vi "TestData_TestAddHash.vi"(8 "error in (no error)":errorcluster caption="错误输入（无错误）", 10 "Record_Text":string, 11 "分隔符(Tab)":string) -> (0 "error out":errorcluster caption="错误输出", 1 "Hash_Code":string, 2 "RecordText Outpout":string, 3 "ok?":bool)   [LabVIEW 2012, in "Lib_UEL.ATE.lvlib" / "Lib_TestData.lvlib"]
uses:
  Lib_TestData.lvlib
  App/Lib_App.lvlib
panel:
  # "功能说明:\n- 添加Hash列\n- 兼容不同的分隔符.\n- 兼容已知的错误格式\n\n\n插入语句标准: 留意转换后最后一列为空.\n- 255列, 以#分隔, \n- 251列, 以#分隔, 缺少: No47记录后,spare1~4列\n- 添加最后一列: hash列"
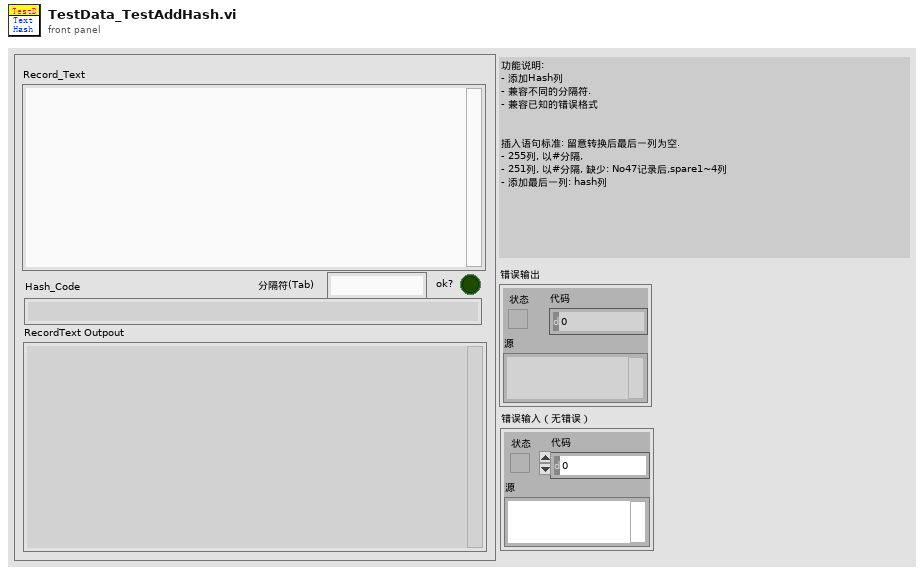
[diagram p1: front panel]
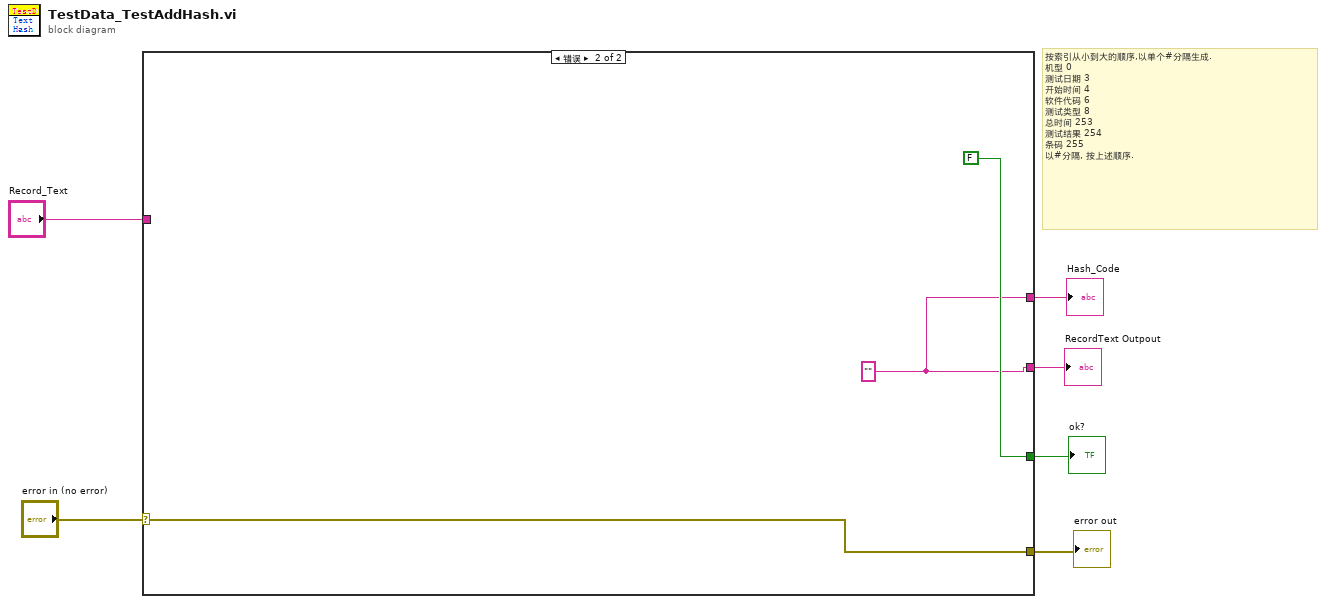
[diagram p0: block diagram]
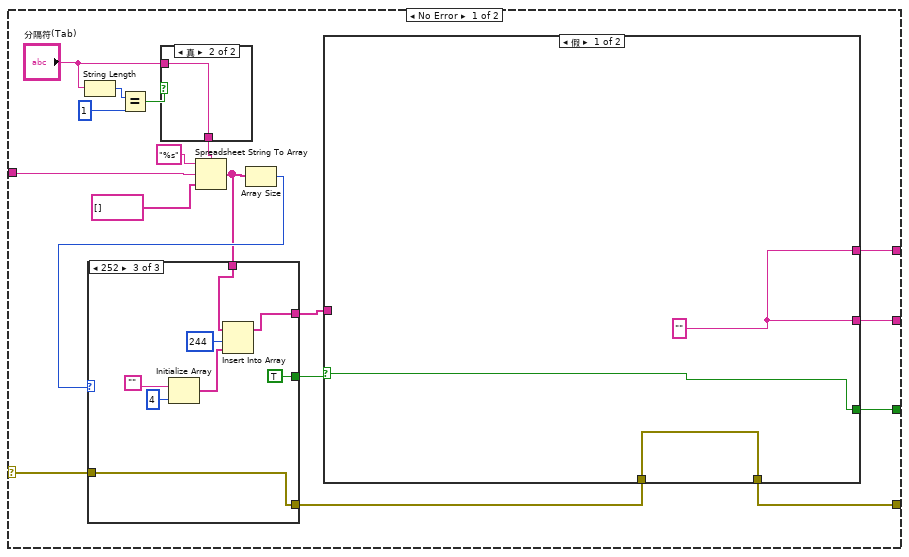
[diagram p2: hidden frame]
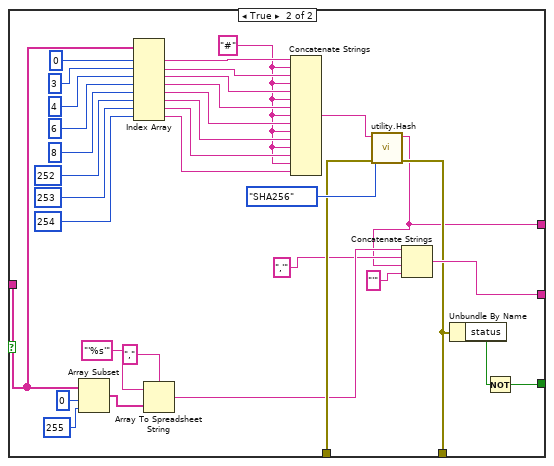
[diagram p3: hidden frame]
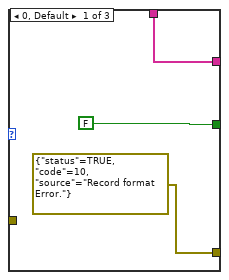
[diagram p4: hidden frame]
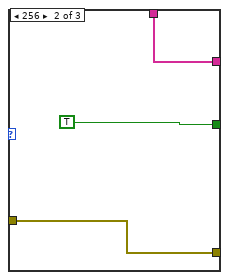
[diagram p5: hidden frame]
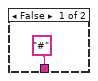
[diagram p6: hidden frame]
diagram:
  # "按索引从小到大的顺序,以单个#分隔生成.\n机型 0\n测试日期 3\n开始时间 4\n软件代码 6\n测试类型 8\n总时间 253\n测试结果 254\n条码 255\n以#分隔, 按上述顺序."
  n1 = case shown="错误" "error in (no error)" {
    selector: "error in (no error)" -> [w12 w80]
    tunnel: [w8 w80] -> w5
    tunnel: [w10 FALSE ("ok?")] -> w4
    tunnel: "Record_Text" -> [w18 _]
    tunnel: [w11 w78] -> w2
    tunnel: [w7 w78] -> w1
    frame No Error {
      n2 = String Length(string="分隔符(Tab)") -> (length=w24:i32)
      n3 = Equal?(x=w24, y=1) -> (x = y?=w22:bool)
      n4 = case shown="真" w22 {
        tunnel: "分隔符(Tab)" -> [_ w77]
        tunnel: ["#" ("分隔符(Tab)") w77] -> w20
        frame False {
        }
        frame True {
        }
      }
      n5 = Spreadsheet String To Array(delimiter (Tab)=w20, format string="%s" ("格式字符串"), spreadsheet string=w18, array type (2D Dbl)=string[] []) -> (array=w13:string[])
      n6 = Array Size(array=w13) -> (size(s)=w16:i32)
      n7 = case shown="252" w16 {
        tunnel: [FALSE TRUE TRUE] -> w15
        tunnel: [w63 w66 w73] -> w14
        tunnel: w13 -> [w63 w66 w74]
        tunnel: [errorcluster {"status"=TRUE, "code"=10, "source"="Record format Error."} ("error IO") w65 w71] -> w9
        tunnel: w12 -> [_ w65 w71]
        frame 0, Default {
        }
        frame 256 {
        }
        frame 252 {
          n8 = Initialize Array("", 4 ("维数大小")) -> (w68:string[])
          n9 = Insert Into Array(array=w74, index=244 ("索引"), new element=w68) -> (w73:string[])
        }
      }
      n10 = case shown="假" w15 {
        selector: w15 -> [w27 _]
        tunnel: w14 -> [_ w57]
        tunnel: [w25 w34] -> w11
        tunnel: [w27 w32] -> w10
        tunnel: w9 -> [w26 w37]
        tunnel: [w26 w33] -> w8
        tunnel: [w25 w28] -> w7
        frame False {
          w25 = "" ("spreadsheet string")
        }
        frame True {
          w40 = "#" ("分隔符(Tab)")
          n11 = Array Subset(array=w57, index=0 ("索引"), length=255 ("长度")) -> (w59:string[])
          n12 = Index Array(array=w57, index #1=0 ("索引"), index #2=3 ("索引"), index #3=4 ("索引"), index #4=6 ("索引"), index #5=8 ("索引"), index #6=252 ("索引"), index #7=253 ("索引"), index #8=254 ("索引")) -> (element #1=w48:string, element #2=w47:string, element #3=w46:string, element #4=w45:string, element #5=w44:string, element #6=w43:string, element #7=w42:string, element #8=w41:string)
          n13 = Array To Spreadsheet String(delimiter (Tab)="," ("分隔符(Tab)"), array=w59, 3:"'%s'" ("格式字符串")) -> (spreadsheet string=w36:string)
          n14 = Concatenate Strings(w48, w40, w47, w40, w46, w40, w45, w40, w44, w40, w43, w40, w42, w40, w41) -> (w39:string)
          n15 = call "utility.Hash.vi"("错误输入（无错误）"=w37, "Hash_Mode"=enum16{"SHA1", "SHA256", "SHA384", "SHA512"}."SHA256", "Input"=w39) -> ("错误输出"=w33:errorcluster, "Hash_Code"=w28:string)  [unwired: 6 in, 1 out]
          n16 = Concatenate Strings(w36, ",'" ("分隔符(Tab)"), w28, "'" ("分隔符(Tab)")) -> (w34:string)
          n17 = Unbundle By Name(w33) -> ("status"=w31:bool)
          n18 = Not(x=w31) -> (.not. x?=w32:bool)
        }
      }
    }
    frame Error {
      w78 = "" ("SQL Outpout")
    }
  }
  "ok?" <- w4
  "RecordText Outpout" <- w2
  "error out" <- w5
  "Hash_Code" <- w1
